vi "DSF.UDP.Transfer.Set Port.vi"(8 "error in (no error)":errorcluster, 10 "Port":u16, 11 "UDP Transfer in":refnum<class "DSF.UDP.Configuration.Transfer.lvclass">) -> (0 "error out":errorcluster, 3 "UDP Transfer out":refnum<class "DSF.UDP.Configuration.Transfer.lvclass">)   [LabVIEW 2016, in "DSF.UDP.Configuration.Transfer.lvclass"]
uses:
  DSF.UDP.Configuration.Transfer.lvclass
  DSF.UDP.Configuration.Transfer.lvclass/DSF.UDP.Configuration.Transfer.ctl
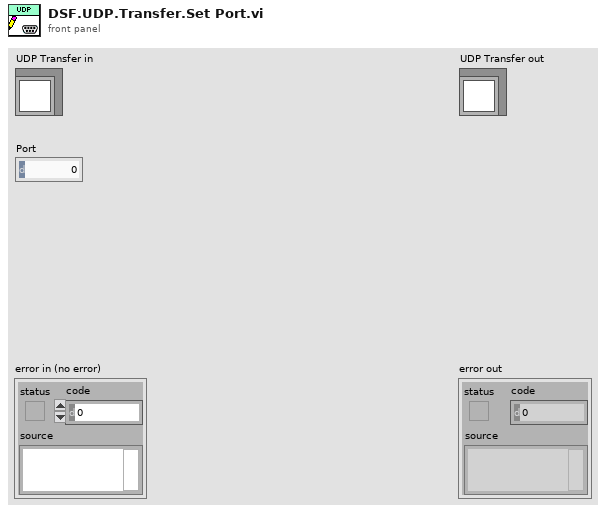
[diagram p1: front panel]
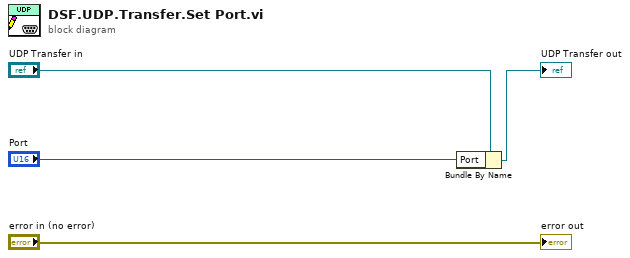
[diagram p0: block diagram]
diagram:
  n1 = Bundle By Name(cluster="UDP Transfer in", "Port"="Port") -> (→"UDP Transfer out":refnum<class "DSF.UDP.Configuration.Transfer.lvclass">)
  "error out" <- "error in (no error)"
